vi "PlanInit.vi"() -> (1 "DataSource Data":string[][](table), 2 "ColumnSetup":T1[](array[typedef]) {"MinWidth" min=2 step=1; "AutoSizeMode" items=["None"=1, "ColumnHeader"=2, "AllCellsExceptHeader"=4, "AllCells"=6, "DisplayedCellsExceptHeader"=8, "DisplayedCells"=10, "Fill"=16]; "FillWeight" min=1 max=100})   [LabVIEW 2020]
uses:
  <vilib>/DataGrid for LabVIEW/source/GridColumn/ColumnDefinition.ctl
  <vilib>/DataGrid for LabVIEW/source/GridColumn/ColumnType.ctl
  <vilib>/DataGrid for LabVIEW/source/GridColumn/GridColumn.lvclass
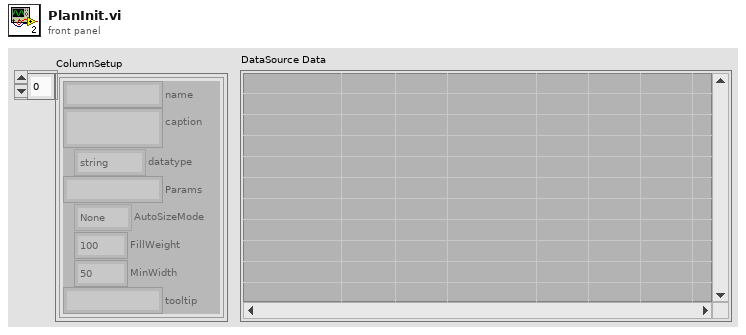
[diagram p1: front panel]
types:
  T1 = typedef "DataGrid.lvlib/GridColumn.lvclass/ColumnDefinition.ctl" = cluster{"name":string, "caption":string, "datatype":T2, "Params":string, "AutoSizeMode":i32, "FillWeight":sgl, "MinWidth":u32, "tooltip":string}
  T2 = typedef "DataGrid.lvlib/GridColumn.lvclass/ColumnType.ctl" = enum16{"string", "image", "check", "numeric", "timestamp", "button", "combo", "link"}
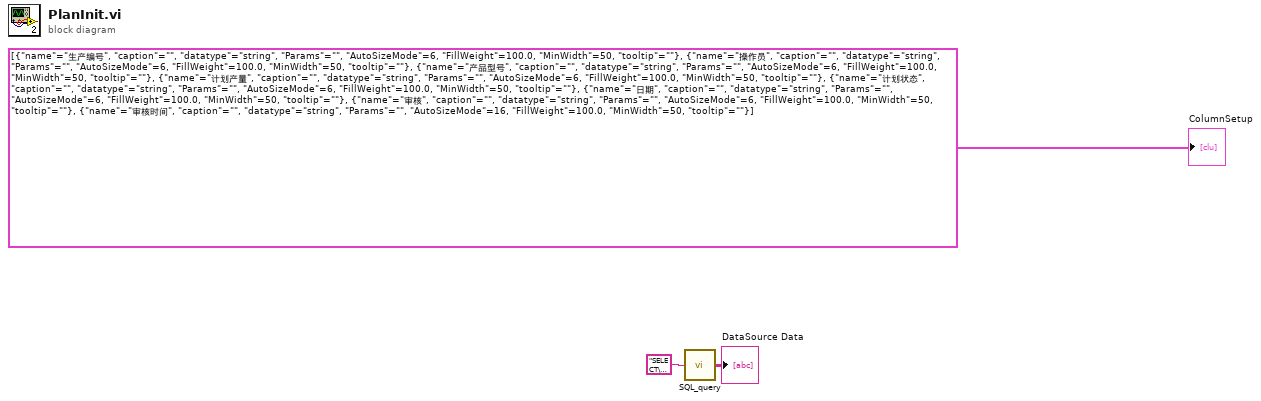
[diagram p0: block diagram]
diagram:
  n1 = call "SQL_query.vi"("SQL query"="SELECT\ndbo.[生产计划].[生产编号],\ndbo.[生产计划].[操作员],\ndbo.[生产计划].[产品型号],\ndbo.[生产计划].[计划产量],\ndbo.[生产计划].[计划状态],\ndbo.[生产计划].[日期],\ndbo.[生产计划].[审核],\ndbo.[生产计划].[审核时间]\n\nFROM\ndbo.[生产计划]\n") -> ("data"=→"DataSource Data":string[][])  [unwired: 3 in, 1 out]
  "ColumnSetup" <- T1[] [{"name"="生产编号", "caption"="", "datatype"=enum."string", "Params"="", "AutoSizeMode"=6, "FillWeight"=100.0, "MinWidth"=50, "tooltip"=""}, {"name"="操作员", "caption"="", "datatype"=enum."string", "Params"="", "AutoSizeMode"=6, "FillWeight"=100.0, "MinWidth"=50, "tooltip"=""}, {"name"="产品型号", "caption"="", "datatype"=enum."string", "Params"="", "AutoSizeMode"=6, "FillWeight"=100.0, "MinWidth"=50, "tooltip"=""}, {"name"="计划产量", "caption"="", "datatype"=enum."string", "Params"="", "AutoSizeMode"=6, "FillWeight"=100.0, "MinWidth"=50, "tooltip"=""}, {"name"="计划状态", "caption"="", "datatype"=enum."string", "Params"="", "AutoSizeMode"=6, "FillWeight"=100.0, "MinWidth"=50, "tooltip"=""}, {"name"="日期", "caption"="", "datatype"=enum."string", "Params"="", "AutoSizeMode"=6, "FillWeight"=100.0, "MinWidth"=50, "tooltip"=""}, {"name"="审核", "caption"="", "datatype"=enum."string", "Params"="", "AutoSizeMode"=6, "FillWeight"=100.0, "MinWidth"=50, "tooltip"=""}, {"name"="审核时间", "caption"="", "datatype"=enum."string", "Params"="", "AutoSizeMode"=16, "FillWeight"=100.0, "MinWidth"=50, "tooltip"=""}] ("ColumnSetup")
